vi "check config property nodes.vi"() -> ()   [LabVIEW 2013, in "CVT Consuming Engine Tests.lvlib"]
uses:
  CVT Consuming Engine Tests.lvlib
  <vilib>/NI/Tag Bus Module Framework/root configuration/Target Types.ctl
  Configuration/CVT Engine Configuration.lvclass
  <vilib>/NI/Configuration Framework/serializable configuration/NISE_CEF_serializable configuration.lvclass/NISE_CEF_serializable configuration.ctl
  <vilib>/NI/Configuration Framework/serializable configuration/NISE_CEF_serializable configuration.lvclass
  <vilib>/NI/Configuration Framework/serializable configuration/Read UID.vi
  <vilib>/NI/Configuration Framework/serializable configuration/get alias.vi
  <vilib>/NI/Configuration Framework/serializable configuration/get view class name.vi
  <vilib>/NI/Tag Bus Module Framework/root configuration/TBM configuration.lvclass
panel:
  out "alias 6":string
  out "error out 6":errorcluster
  out "execution class name 5":string
  out "error out 5":errorcluster
  out "instances allowed 4":i32
  out "error out 4":errorcluster
  out "UID 3":string
  out "error out 3":errorcluster
  out "view class name 2":string
  out "error out 2":errorcluster
  out "supported targets":T1[](array[typedef])
  out "error out":errorcluster
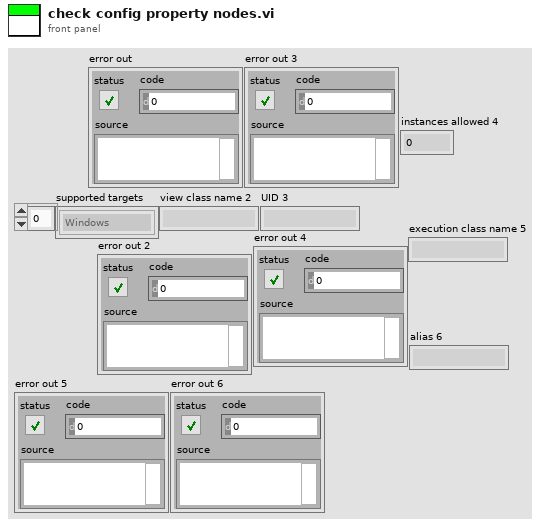
[diagram p1: front panel]
types:
  T1 = typedef "TBM configuration.lvclass/Target Types.ctl" = enum16{"Windows", "Mac", "Linux", "Linux RT ARM", "VxWorks", "Pharlap", "Other", "Linux RT x64"}
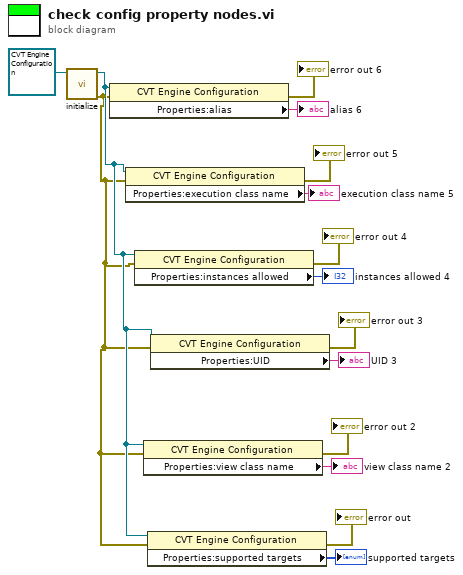
[diagram p0: block diagram]
diagram:
  n1 = call-dynamic "initialize.vi"("configuration in"=refnum<class "CVT Engine Configuration.lvclass"> refnum ("CVT Engine Configuration")) -> ("error out"=w13:errorcluster, "configuration out"=w14:refnum<class "CVT Engine Configuration.lvclass">)  [unwired: 8 in, 1 out]
  n2 = property class="CVT Engine Configuration"(reference=w14, error in=w13) -> (error out=→"error out 6":errorcluster, "Properties:alias"=→"alias 6":string)  [unwired: 1 out]
  n3 = property class="CVT Engine Configuration"(reference=w14, error in=w13) -> (error out=→"error out 5":errorcluster, "Properties:execution class name"=→"execution class name 5":string)  [unwired: 1 out]
  n4 = property class="CVT Engine Configuration"(reference=w14, error in=w13) -> (error out=→"error out 4":errorcluster, "Properties:instances allowed"=→"instances allowed 4":i32)  [unwired: 1 out]
  n5 = property class="CVT Engine Configuration"(reference=w14, error in=w13) -> (error out=→"error out 2":errorcluster, "Properties:view class name"=→"view class name 2":string)  [unwired: 1 out]
  n6 = property class="CVT Engine Configuration"(reference=w14, error in=w13) -> (error out=→"error out":errorcluster, "Properties:supported targets"=→"supported targets":T1[])  [unwired: 1 out]
  n7 = property class="CVT Engine Configuration"(reference=w14, error in=w13) -> (error out=→"error out 3":errorcluster, "Properties:UID"=→"UID 3":string)  [unwired: 1 out]
